vi "final_phd_1.vi"() -> ()   [LabVIEW 2024]
uses:
  <vilib>/Analysis/baseanly.llb/Mean (DBL).vi
  <vilib>/Instr/_visa.llb/VISA Configure Serial Port (Instr).vi
  <vilib>/measure/maspectr.llb/FFT Power Spectrum and PSD for 1 Chan.vi
  <vilib>/Analysis/NI_AALBase.lvlib
  <vilib>/measure/NI_MAPro.lvlib
panel:
  out "Waveform Graph":dbl[](graph)
  out "AI output":u8[](array[numeric])
  in  "Timeout":u32=100
  in  "default name":string
  in  "number":i32=10
  out "Waveform Graph 3":cluster{"f0":dbl, "df":dbl, "magnitude":dbl[]}(graph)={"f0"=0.0, "df"=inf, "magnitude"=[]}
  in  "Signals":waveform(dbl)={"t0"=timestamp(0 s since 1904-01-01), "dt"=0.01, "Y"=[]}
  in  "low cutoff freq":dbl=40.0 format="%0.2f"
  in  "Filter":bool
  in  "Pulse cycle":dbl=1.0
  out "?":dbl(graph)=nan
  in  "milliseconds to wait":u32
  in  "Add Wave 2":bool
  out "Save Status":bool
  in  "Save":bool caption="Save Process"
  out "str_ai_output":string="N.A"
  out "num_sensor_sam_per_cycle":u32=333 caption="Samples/Cycle"
  in  "cbx_sensor_sam_rate":string(combo)="66667" caption="Sample Rate (Hz)"
  in  "num_pulse_samples":u32=500 caption="Samples" max=10000 step=100
  in  "Hidden Controls":T1(tab)
  out "timeout_for_small_data":u32=1000
  out "baud rate":u32=115200
  out "timeout_default":u32=50
  out "termination char":u8
  out "CMD_ID_GET":string
  out "CMD_ID_RUN":string
  out "CMD_ID_NONE":string
  out "CMD_ID_SET":string
  out "CMD_RUN_NONE":string
  out "CMD_RUN_START":string
  out "CMD_RUN_STOP":string
  out "PG_PULSE_NONE":string
  out "PG_PULSE_SQUARE":string
  out "PG_PULSE_SINE":string
  out "RESPONSE_LEN":u32=48
  out "TIM_FREQ":u32=64000000
  out "has_response":bool
  out "ADC_CONVERSION_CYCLES":dbl=8.5
  out "ADC_FREQ":u32=64000000
  out "ADC_SAMPLING_TIME":dbl[](array[numeric])=[2.5, 6.5, 12.5, 24.5, 47.5, 92.5, 247.5, 640.5]
  out "ADC_CLOCK_PRESCALER":u32[](array[numeric])=[1, 2, 4, 6, 8, 10, 12, 16, 32, 64, 128, 256]
  out "sam_rates":cluster{u32, u32, dbl}[](array[cluster])=[{385, 256, 640.5}, {770, 128, 640.5}, {977, 256, 247.5}, {1541, 64, 640.5}, {1953, 128, 247.5}, {2475, 256, 92.5}, {3082, 32, 640.5}, {3906, 64, 247.5}, {4464, 256, 47.5}, {4950, 128, 92.5}, {6163, 16, 640.5}, {7576, 256, 24.5}, {7812, 32, 247.5}, {8218, 12, 640.5}, {8929, 128, 47.5}, {9861, 10, 640.5}, {9901, 64, 92.5}, {11905, 256, 12.5}, {12327, 8, 640.5}, {15152, 128, 24.5}, {15625, 16, 247.5}, {16436, 6, 640.5}, {16667, 256, 6.5}, {17857, 64, 47.5}, {19802, 32, 92.5}, {20833, 12, 247.5}, {22727, 256, 2.5}, {23810, 128, 12.5}, {24653, 4, 640.5}, {25000, 10, 247.5}, {30303, 64, 24.5}, {31250, 8, 247.5}, {33333, 128, 6.5}, {35714, 32, 47.5}, {39604, 16, 92.5}, {41667, 6, 247.5}, {45455, 128, 2.5}, {47619, 64, 12.5}, {49307, 2, 640.5}, {52805, 12, 92.5}, {60606, 32, 24.5}, {62500, 4, 247.5}, {63366, 10, 92.5}, {66667, 64, 6.5}, {71429, 16, 47.5}, {79208, 8, 92.5}, {90909, 64, 2.5}, {95238, 12, 47.5}, {95238, 32, 12.5}, {98613, 1, 640.5}, {105611, 6, 92.5}, {114286, 10, 47.5}, {121212, 16, 24.5}, {125000, 2, 247.5}, {133333, 32, 6.5}, {142857, 8, 47.5}, {158416, 4, 92.5}, {161616, 12, 24.5}, {181818, 32, 2.5}, {190476, 6, 47.5}, {190476, 16, 12.5}, {193939, 10, 24.5}, {242424, 8, 24.5}, {250000, 1, 247.5}, {253968, 12, 12.5}, {266667, 16, 6.5}, {285714, 4, 47.5}, {304762, 10, 12.5}, {316832, 2, 92.5}, {323232, 6, 24.5}, {355556, 12, 6.5}, {363636, 16, 2.5}, {380952, 8, 12.5}, {426667, 10, 6.5}, {484848, 4, 24.5}, {484848, 12, 2.5}, {507937, 6, 12.5}, {533333, 8, 6.5}, {571429, 2, 47.5}, {581818, 10, 2.5}, {633663, 1, 92.5}, {711111, 6, 6.5}, {727273, 8, 2.5}, {761905, 4, 12.5}, {969697, 2, 24.5}, {969697, 6, 2.5}, {1066667, 4, 6.5}, {1142857, 1, 47.5}, {1454545, 4, 2.5}, {1523810, 2, 12.5}, {1939394, 1, 24.5}, {2133333, 2, 6.5}, {2909091, 2, 2.5}, {3047619, 1, 12.5}, {4266667, 1, 6.5}, {5818182, 1, 2.5}]
  out "cbx_sensor_sam_rate_sel_idx":u32=43
  in  "num_senor_read_samples":u32=333 caption="Read Samples" max=10000 step=100
  in  "num_pulse_min_val":dbl caption="Minimum Value (V)" min=0.0 max=1.0 step=0.1
  in  "num_pulse_dutyc":u32=50 caption="Duty Cycle (%)" max=100 step=10
  in  "num_pulse_max_val":dbl=3.0 caption="Maximum Value (V)" min=0.0 max=3.3 step=0.1
  out "?":string
  in  "btn_get":bool
  in  "cbx_pulse_type":string(combo)="1" caption="Type"
  in  "num_pulse_freq":u32=200 caption="Frequency (Hz)" max=2000 step=100
  in  "btn_set":bool
  in  "btn_start_stop":bool
  in  "VISA resource name":refnum<visa-resource-name>="COM10"
  out "read buffer":string
  out "Sensor Signal":dbl[](graph)
  # "NDT COMPACT SYSTEM"
  # "AI Output"
  # "Write Buffer"
  # "Functions Adjustment"
  # "Read Buffer"
  # "Communication"
  # "Settings"
  # "Pulse"
  # "AI OUTPUT"
  # "Sensor"
  # "CT38_koma"
  # "SS400"
  # "Inox201"
  # "Inox304"
  # "Inox316"
  # "AL5052"
  # "Air"
  # "Save data"
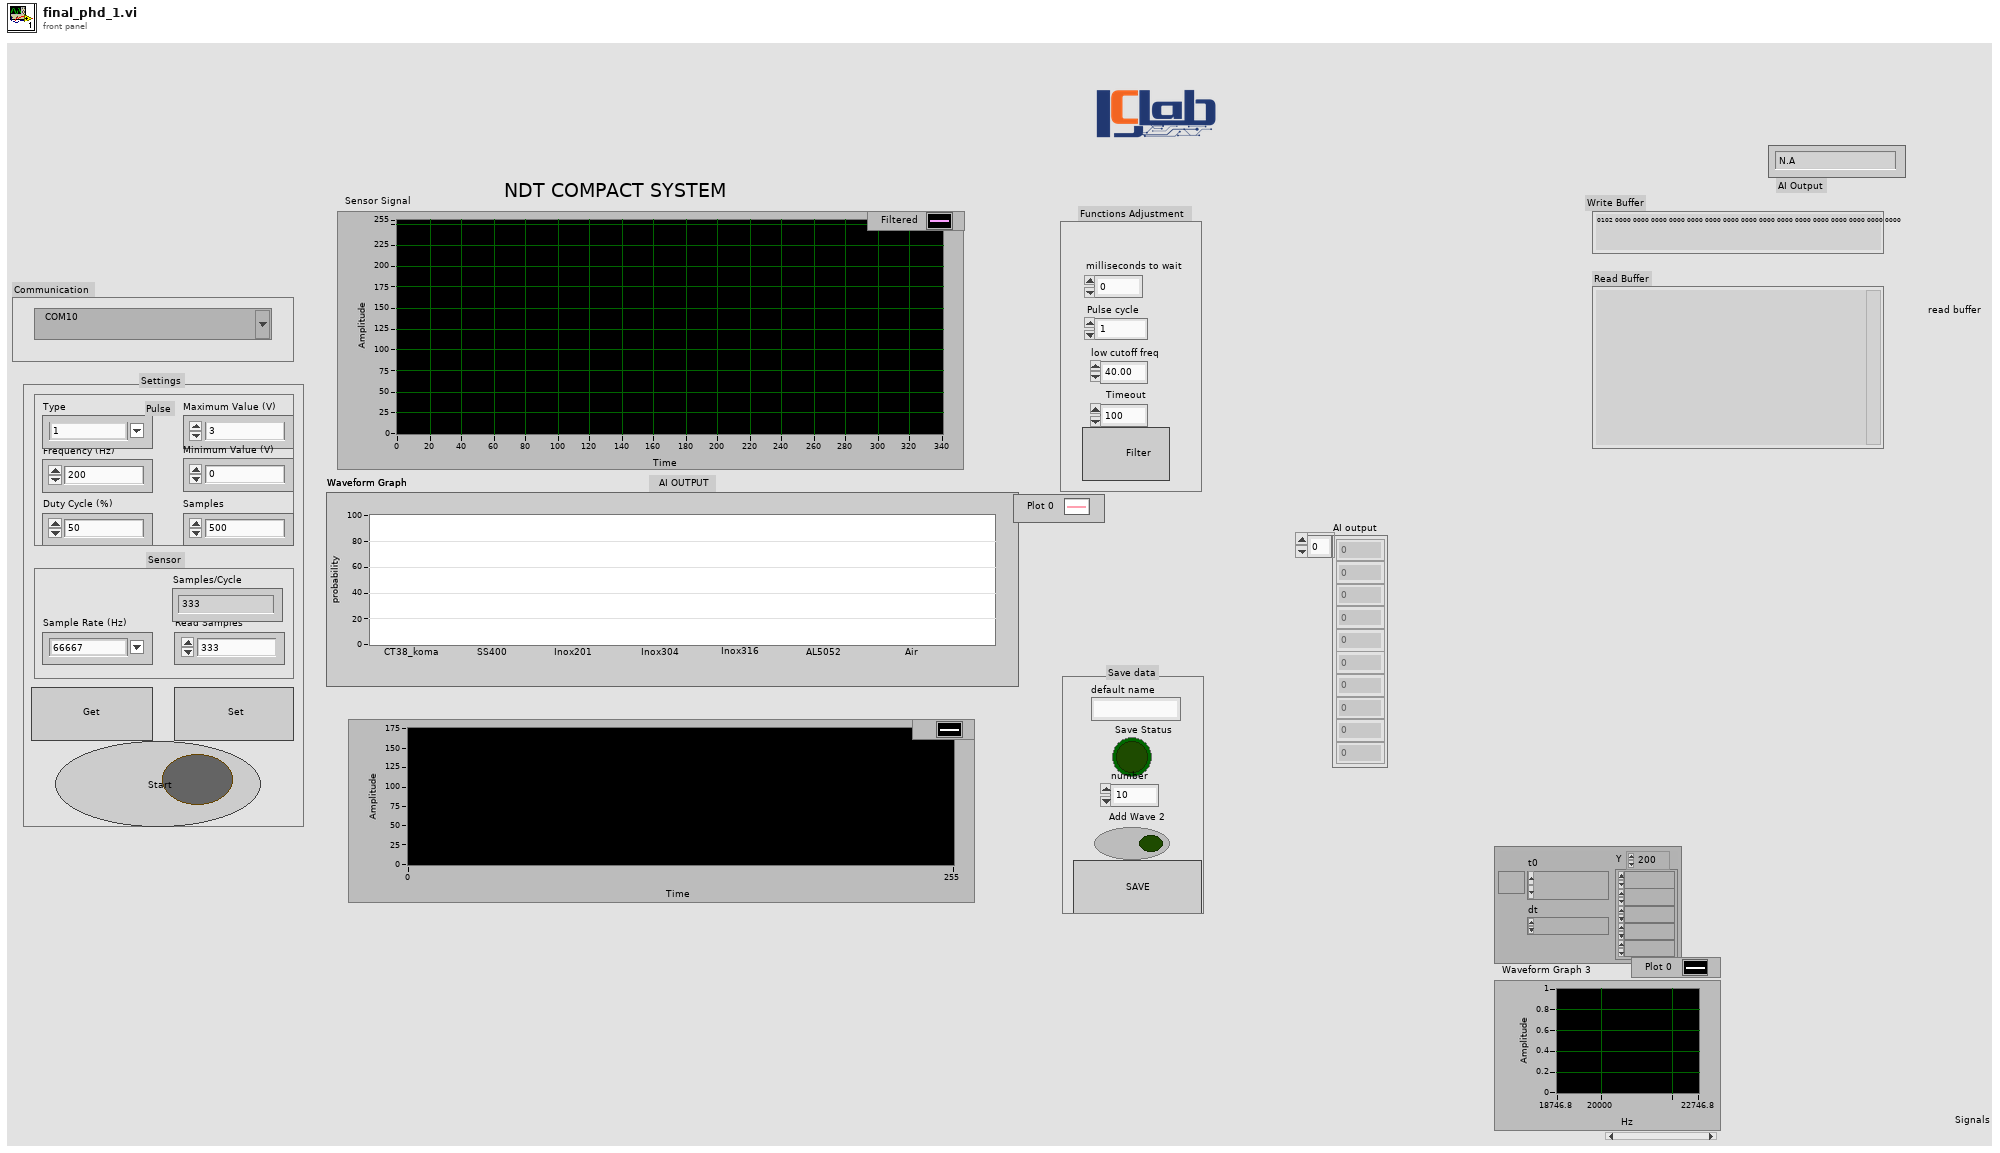
[diagram p1: front panel]
types:
  T1 = enum32{"Page 1", "Page 2", "Page 3", "Page 4", "Page 5"}
  T2 = enum8{"Enabled", "Disabled", "Disabled and Grayed Out"}
  T3 = enum16{"big-endian, network order", "native, host order", "little-endian"}
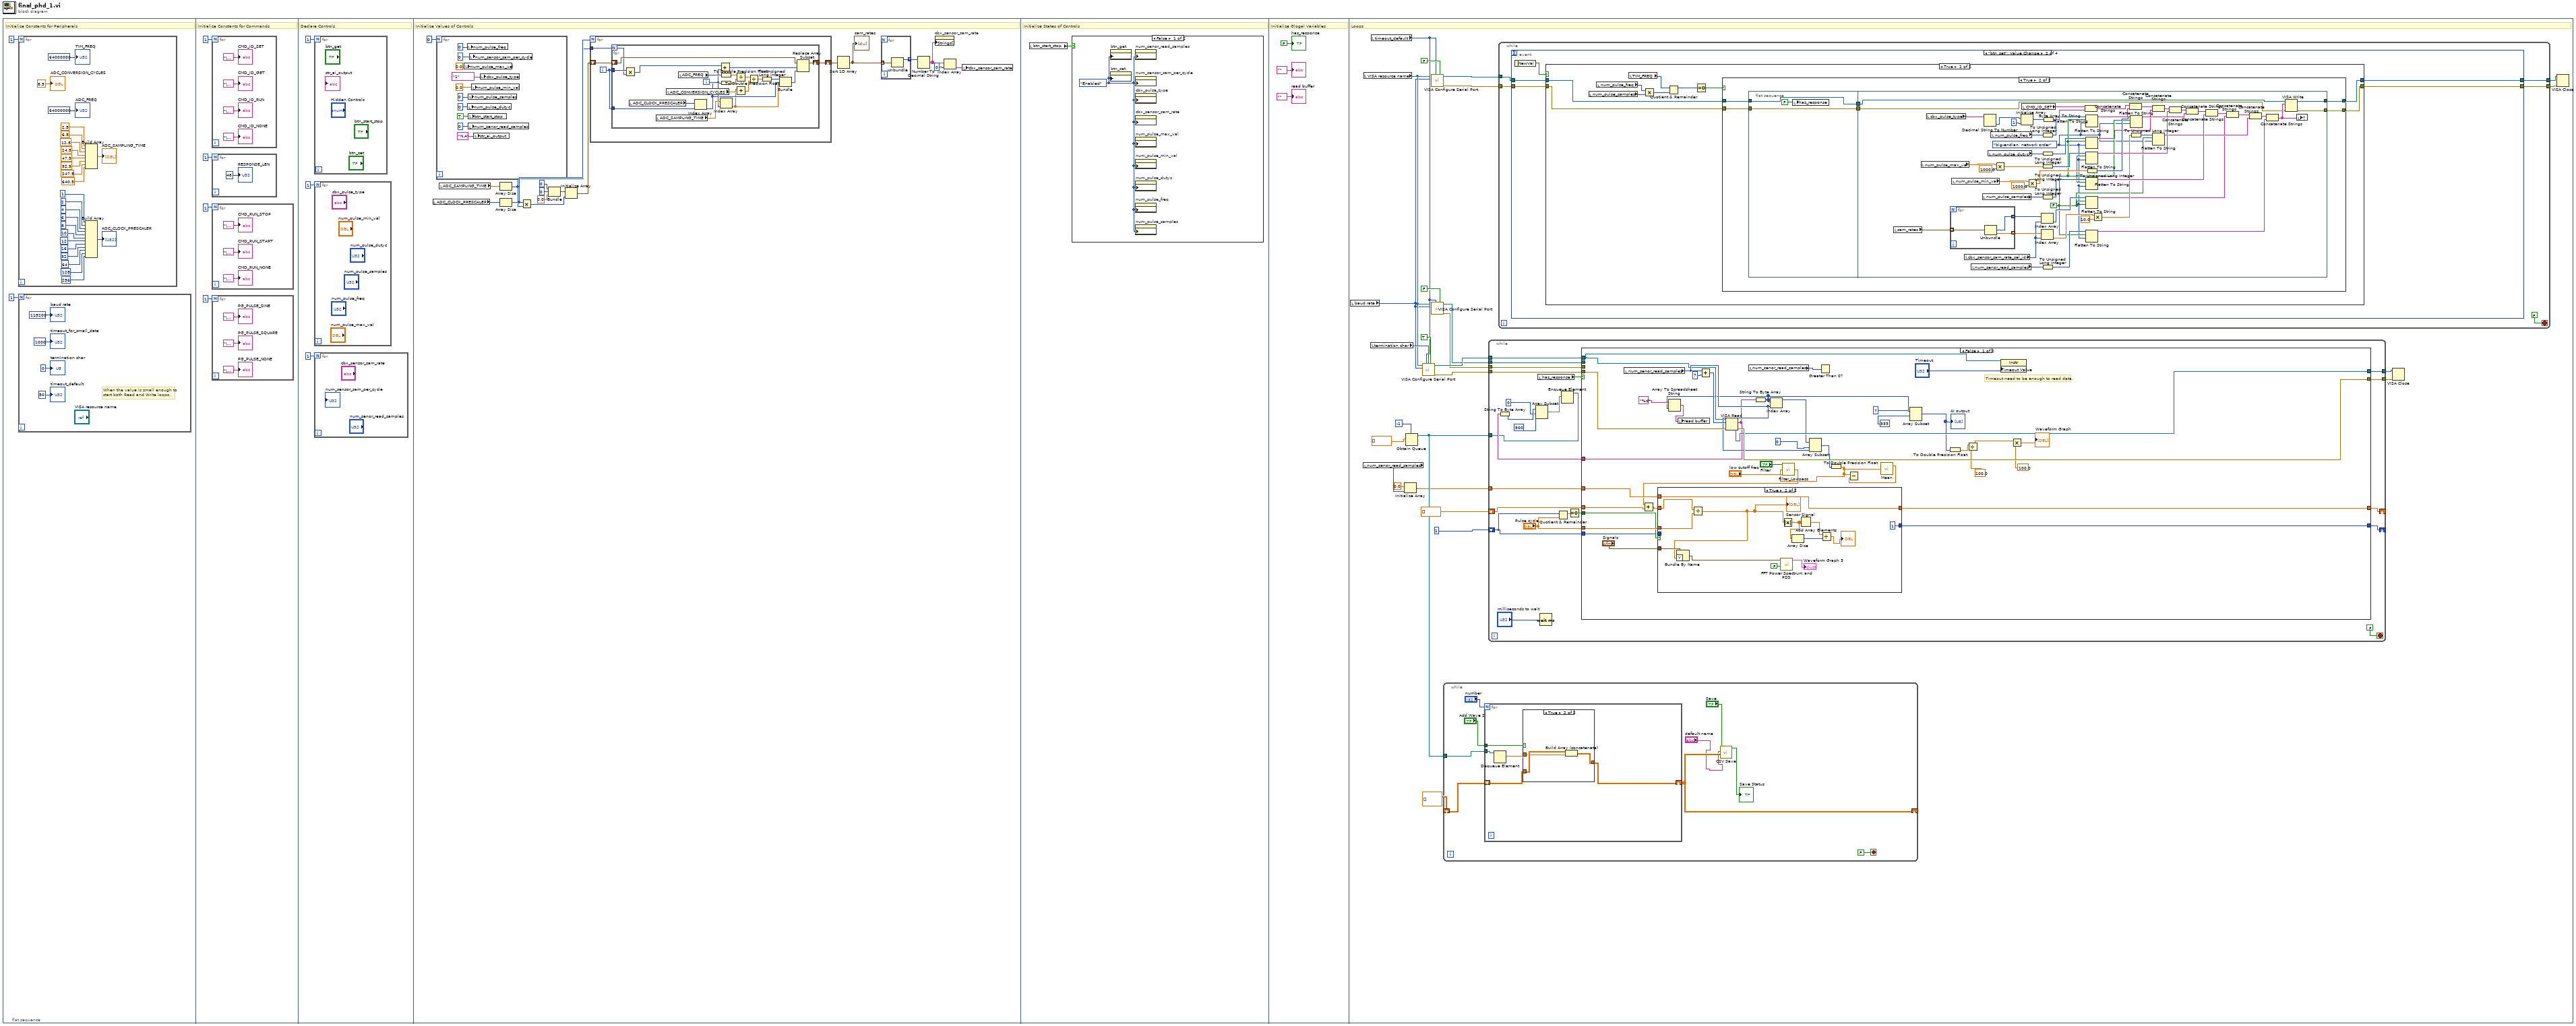
[diagram p0: block diagram]
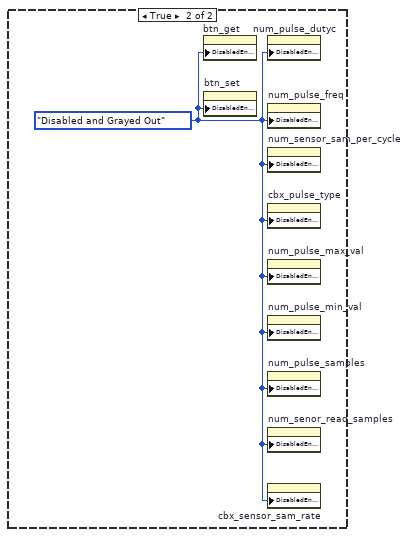
[diagram p2: hidden frame]
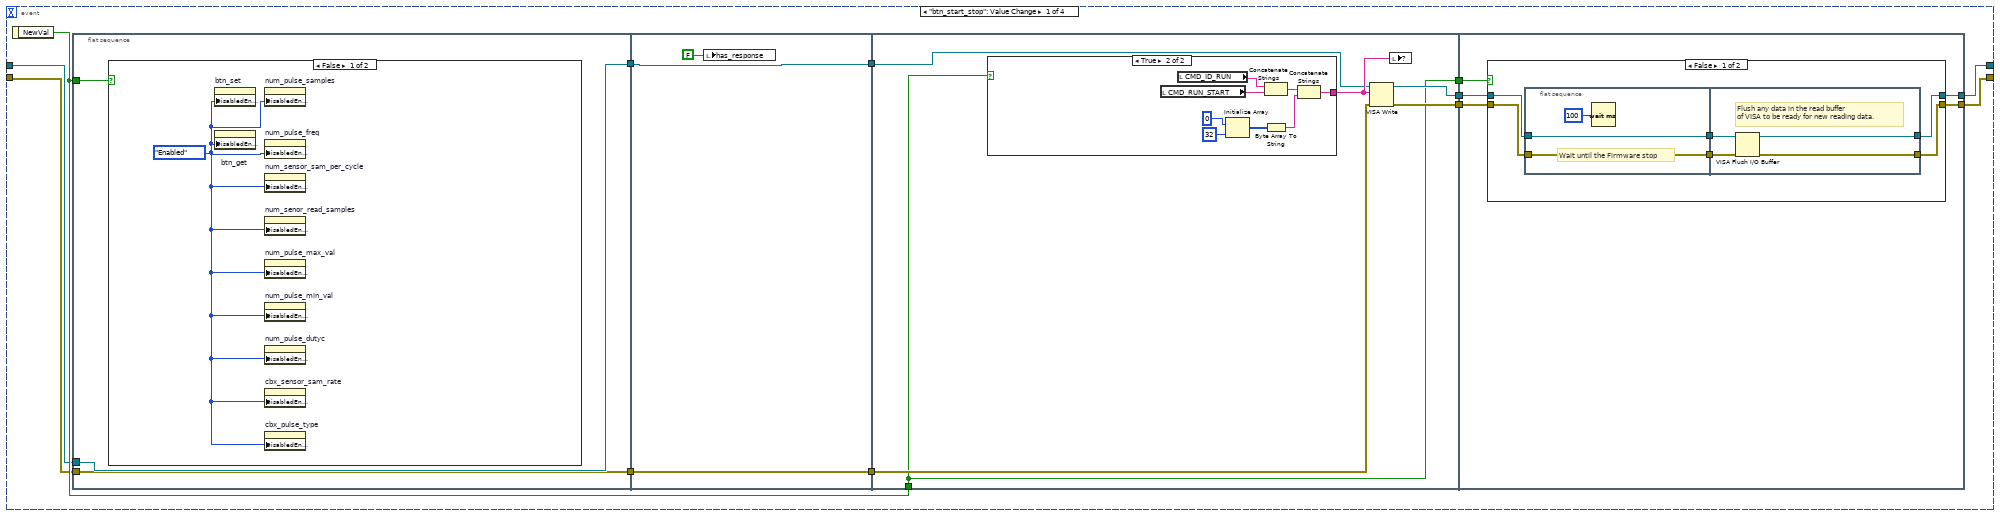
[diagram p4: hidden frame]
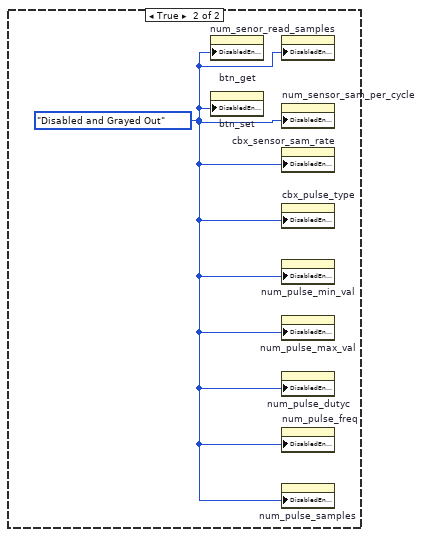
[diagram p5: hidden frame]
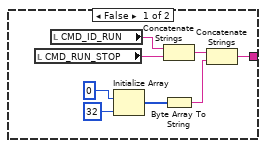
[diagram p6: hidden frame]
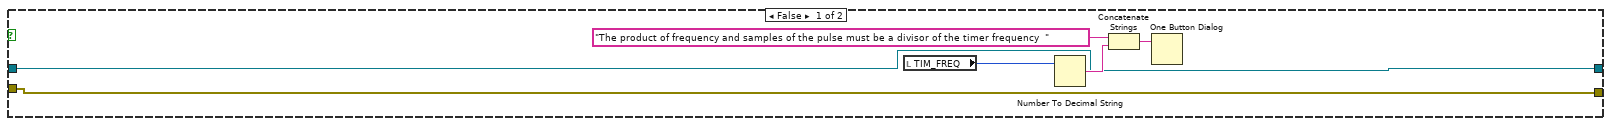
[diagram p9: hidden frame]
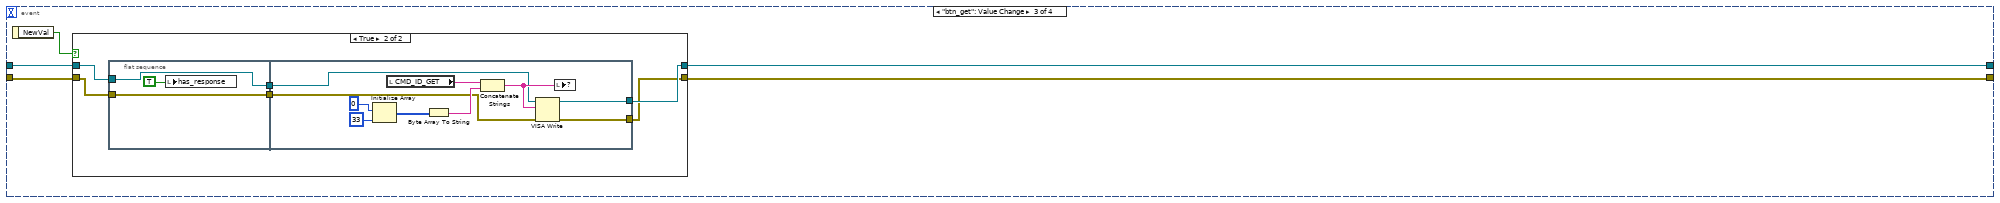
[diagram p10: hidden frame]
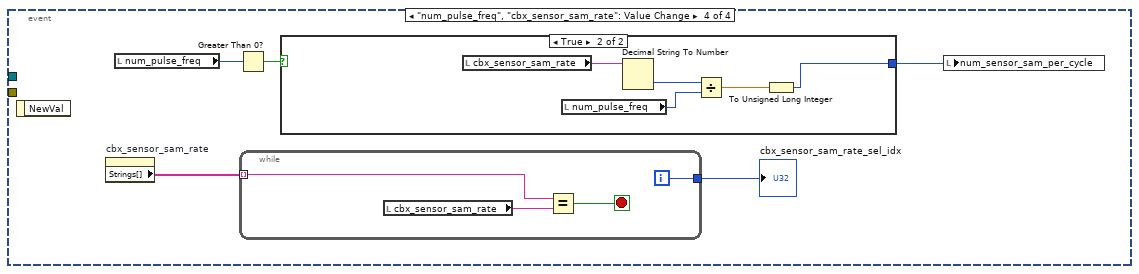
[diagram p12: hidden frame]
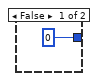
[diagram p13: hidden frame]
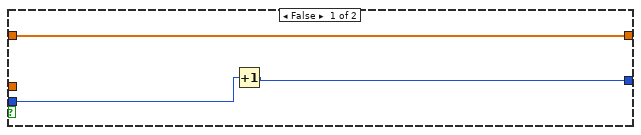
[diagram p14: hidden frame]
diagram:
  n1 = flat-sequence {
    frame #0 {
      # "Initialize Constants for Peripherals"
      n2 = for {
        N: 1 -> [_]
        n3 = Build Array(2.5 ("element"), 6.5 ("element"), 12.5 ("element"), 24.5 ("element"), 47.5 ("element"), 92.5 ("element"), 247.5 ("element"), 640.5 ("element")) -> (→"ADC_SAMPLING_TIME":dbl[])
        n4 = Build Array(u32 1 ("element"), u32 2 ("element"), u32 4 ("element"), u32 6 ("element"), u32 8 ("element"), u32 10 ("element"), u32 12 ("element"), u32 16 ("element"), u32 32 ("element"), u32 64 ("element"), u32 128 ("element"), u32 256 ("element")) -> (→"ADC_CLOCK_PRESCALER":u32[])
        "ADC_CONVERSION_CYCLES" <- 8.5
        "ADC_FREQ" <- 64000000
        "TIM_FREQ" <- 64000000
      }
      n5 = for {
        N: 1 -> [_]
        # "When the value is small enough to\nstart both Read and Write loops."
        "baud rate" <- u32 115200 ("baud rate (9600)")
        "timeout_default" <- u32 50 ("timeout (10sec)")
        "termination char" <- u8 0 ("termination char\n(0xA = '\\n' = LF)")
        "timeout_for_small_data" <- u32 1000 ("timeout_default 2")
      }
    }
    frame #1 {
      # "Initialize Constants for Commands"
      n6 = for {
        N: 1 -> [_]
        "CMD_ID_NONE" <- "\u0000"
        "CMD_ID_RUN" <- "\u0001"
        "CMD_ID_GET" <- "\u0002"
        "CMD_ID_SET" <- "\u0003"
      }
      n7 = for {
        N: 1 -> [_]
        "RESPONSE_LEN" <- 48
      }
      n8 = for {
        N: 1 -> [_]
        "CMD_RUN_NONE" <- "\u0000"
        "CMD_RUN_START" <- "\u0001"
        "CMD_RUN_STOP" <- "\u0002"
      }
      n9 = for {
        N: 1 -> [_]
        "PG_PULSE_NONE" <- "\u0000"
        "PG_PULSE_SQUARE" <- "\u0001"
        "PG_PULSE_SINE" <- "\u0002"
      }
    }
    frame #2 {
      # "Declare Controls"
      n10 = for {
        N: 1 -> [_]
      }
      n11 = for {
        N: 1 -> [_]
      }
      n12 = for {
        N: 1 -> [_]
      }
    }
    frame #3 {
      # "Initialize Values of Controls"
      n13 = local read "ADC_CLOCK_PRESCALER"() -> (w60:u32[])
      n14 = for {
        N: 0 -> [_]
        n15 = local write "num_pulse_max_val"(0.0 ("num_pulse_amp")) -> ()
        n16 = local write "num_pulse_freq"(u32 0 ("num_pulse_freq")) -> ()
        n17 = local write "num_pulse_dutyc"(u32 0 ("num_pulse_dutyc")) -> ()
        n18 = local write "num_pulse_samples"(u32 0 ("num_pulse_samples")) -> ()
        n19 = local write "btn_start_stop"(TRUE ("btn_start_stop")) -> ()
        n20 = local write "num_senor_read_samples"(u32 0 ("num_read_samples")) -> ()
        n21 = local write "num_sensor_sam_per_cycle"(u32 0 ("num_sensor_sam_per_cycle")) -> ()
        n22 = local write "num_pulse_min_val"(0.0 ("num_pulse_amp_offset")) -> ()
        n23 = local write "str_ai_output"("N.A" ("str_ai_result")) -> ()
        n24 = local write "cbx_pulse_type"("1" ("cbx_pulse_type")) -> ()
      }
      n25 = local read "ADC_SAMPLING_TIME"() -> (w59:dbl[])
      n26 = Array Size(array=w59) -> (size(s)=w55:i32)
      n27 = Array Size(array=w60) -> (size(s)=w56:i32)
      n28 = Multiply(x=w56, y=w55) -> (x*y=w57:i32)
      n29 = Bundle(u32 0, u32 0, 0.0) -> (w61:cluster{u32, u32, dbl})  [unwired: 1 in]
      n30 = Initialize Array(w61, w57) -> (w54:cluster{u32, u32, dbl}[])
      n31 = for {
        N: w56 -> [_]
        tunnel: w55 -> [w72]
        shift-right: [w70] -> w58
        shift-left: w54 -> [w71]
        i -> [w69]
        n32 = for {
          N: w72 -> [w81]
          tunnel: w69 -> [w90]
          shift-right: [w78] -> w70
          shift-left: w71 -> [w84]
          tunnel: w69 -> [w82]
          i -> [w80]
          n33 = Multiply(x=w82, y=w81) -> (x*y=w83:i32)
          n34 = local read "ADC_CLOCK_PRESCALER"() -> (w91:u32[])
          n35 = local read "ADC_SAMPLING_TIME"() -> (w92:dbl[])
          n36 = local read "ADC_CONVERSION_CYCLES"() -> (w93:dbl)
          n37 = local read "ADC_FREQ"() -> (w86:u32)
          n38 = Index Array(array=w91, index=w90) -> (element=w74:u32)
          n39 = Add(x=w83, y=w80) -> (x+y=w79:i32)
          n40 = To Double Precision Float(number=w86) -> (double precision float=w85:dbl)
          n41 = To Double Precision Float(number=w74) -> (double precision float=w87:dbl)
          n42 = Index Array(array=w92, index=w80) -> (element=w73:dbl)
          n43 = Divide(x=w85, y=w87) -> (x/y=w89:dbl)
          n44 = Add(x=w93, y=w73) -> (x+y=w88:dbl)
          n45 = Divide(x=w89, y=w88) -> (x/y=w76:dbl)
          n46 = To Unsigned Long Integer(number=w76) -> (unsigned 32bit integer=w75:u32)
          n47 = Bundle(w75, "element"=w74, "element"=w73) -> (w77:cluster{u32, "element":u32, "element":dbl})  [unwired: 1 in]
          n48 = Replace Array Subset(array=w84, new element=w77, index=w79) -> (w78:cluster{u32, u32, dbl}[])
        }
      }
      n49 = Sort 1D Array(array=w58) -> (sorted array=w62:cluster{u32, u32, dbl}[])
      "sam_rates" <- w62
      n50 = for {
        tunnel: w62 -> [w68] mode=indexing
        tunnel: [w67] -> w63 mode=indexing
        n51 = Unbundle(w68) -> (w67:u32)  [unwired: 2 out]
      }
      n52 = Number To Decimal String(number=w63) -> (decimal integer string=w64:string[])  [unwired: 1 in]
      n53 = property on="cbx_sensor_sam_rate" class="CmbBox"("Strings[]"=w64) -> ()  [unwired: 2 in, 2 out]
      n54 = Index Array(array=w64, index=0) -> (element=w65:string)
      n55 = local write "cbx_sensor_sam_rate"(w65) -> ()
    }
    frame #4 {
      # "Initialize States of Controls"
      n56 = local read "btn_start_stop"() -> (w104:bool)
      n57 = case shown="False" w104 {
        frame False {
          w105 = T2."Enabled" ("Disabled")
          n58 = property on="btn_get" class="Bool (strict)"("DisabledEnum"=w105) -> ()  [unwired: 2 in, 2 out]
          n59 = property on="btn_set" class="Bool (strict)"("DisabledEnum"=w105) -> ()  [unwired: 2 in, 2 out]
          n60 = property on="num_senor_read_samples" class="DigNum (strict)"("DisabledEnum"=w105) -> ()  [unwired: 2 in, 2 out]
          n61 = property on="num_sensor_sam_per_cycle" class="DigNum (strict)"("DisabledEnum"=w105) -> ()  [unwired: 2 in, 2 out]
          n62 = property on="cbx_pulse_type" class="CmbBox"("DisabledEnum"=w105) -> ()  [unwired: 2 in, 2 out]
          n63 = property on="cbx_sensor_sam_rate" class="CmbBox"("DisabledEnum"=w105) -> ()  [unwired: 2 in, 2 out]
          n64 = property on="num_pulse_max_val" class="DigNum (strict)"("DisabledEnum"=w105) -> ()  [unwired: 2 in, 2 out]
          n65 = property on="num_pulse_min_val" class="DigNum (strict)"("DisabledEnum"=w105) -> ()  [unwired: 2 in, 2 out]
          n66 = property on="num_pulse_dutyc" class="DigNum (strict)"("DisabledEnum"=w105) -> ()  [unwired: 2 in, 2 out]
          n67 = property on="num_pulse_freq" class="DigNum (strict)"("DisabledEnum"=w105) -> ()  [unwired: 2 in, 2 out]
          n68 = property on="num_pulse_samples" class="DigNum (strict)"("DisabledEnum"=w105) -> ()  [unwired: 2 in, 2 out]
        }
        frame True {
          w106 = T2."Disabled and Grayed Out" ("Disabled")
          n69 = property on="btn_get" class="Bool (strict)"("DisabledEnum"=w106) -> ()  [unwired: 2 in, 2 out]
          n70 = property on="btn_set" class="Bool (strict)"("DisabledEnum"=w106) -> ()  [unwired: 2 in, 2 out]
          n71 = property on="num_pulse_dutyc" class="DigNum (strict)"("DisabledEnum"=w106) -> ()  [unwired: 2 in, 2 out]
          n72 = property on="num_pulse_freq" class="DigNum (strict)"("DisabledEnum"=w106) -> ()  [unwired: 2 in, 2 out]
          n73 = property on="num_sensor_sam_per_cycle" class="DigNum (strict)"("DisabledEnum"=w106) -> ()  [unwired: 2 in, 2 out]
          n74 = property on="cbx_pulse_type" class="CmbBox"("DisabledEnum"=w106) -> ()  [unwired: 2 in, 2 out]
          n75 = property on="num_pulse_max_val" class="DigNum (strict)"("DisabledEnum"=w106) -> ()  [unwired: 2 in, 2 out]
          n76 = property on="num_pulse_min_val" class="DigNum (strict)"("DisabledEnum"=w106) -> ()  [unwired: 2 in, 2 out]
          n77 = property on="num_pulse_samples" class="DigNum (strict)"("DisabledEnum"=w106) -> ()  [unwired: 2 in, 2 out]
          n78 = property on="num_senor_read_samples" class="DigNum (strict)"("DisabledEnum"=w106) -> ()  [unwired: 2 in, 2 out]
          n79 = property on="cbx_sensor_sam_rate" class="CmbBox"("DisabledEnum"=w106) -> ()  [unwired: 2 in, 2 out]
        }
      }
    }
    frame #5 {
      # "Initialize Glogal Variables"
      "?" <- "" ("write buffer")
      "read buffer" <- "" ("read buffer")
      "has_response" <- FALSE
    }
    frame #6 {
      # "Loops"
      n80 = local read "baud rate"() -> (w119:u32)
      n81 = local read "num_senor_read_samples"() -> (w112:u32)
      n82 = local read "VISA resource name"() -> (w120:refnum<visa-resource-name>)
      n83 = local read "termination char"() -> (w132:u8)
      n84 = local read "timeout_default"() -> (w121:u32)
      n85 = Initialize Array(0.0 ("element"), w112) -> (w111:dbl[])
      n86 = Obtain Queue(max queue size (-1, unlimited)=-1, element data type=dbl[] []) -> (queue out=w116:refnum<queue>)  [unwired: 3 in, 2 out]
      n87 = call-poly "VISA Configure Serial Port"("VISA resource name"=w120, "timeout (10sec)"=w121, "termination char\n(0xA = '\\n' = LF)"=w132, "Enable Termination\nChar (T)"=TRUE ("Enable Termination\nChar (T)"), "baud rate (9600)"=w119) -> ("VISA resource name out"=w133:refnum<visa-resource-name>, "error out"=w127:errorcluster)  [unwired: 9 in]
      n88 = call-poly "VISA Configure Serial Port"("VISA resource name"=w120, "timeout (10sec)"=w121, "Enable Termination\nChar (T)"=FALSE ("Enable Termination\nChar (T)"), "baud rate (9600)"=w119) -> ("VISA resource name out"=w124:refnum<visa-resource-name>, "error out"=w123:errorcluster)  [unwired: 10 in]
      n89 = call-poly "VISA Configure Serial Port"("VISA resource name"=w120, "timeout (10sec)"=w121, "Enable Termination\nChar (T)"=FALSE ("Enable Termination\nChar (T)"), "baud rate (9600)"=w119) -> ("VISA resource name out"=w125:refnum<visa-resource-name>, "error out"=w126:errorcluster)  [unwired: 10 in]
      n90 = while {
        tunnel: w116 -> [w142]
        shift-right: [w139] -> _
        shift-left: dbl[][] [] -> [w140]
        stop <- FALSE stop-if-true
        n91 = for {
          N: "number" -> [_]
          tunnel: "Add Wave 2" -> [w149]
          shift-right: [w145] -> w139
          shift-left: w140 -> [w148]
          tunnel: w142 -> [w147]
          n92 = Dequeue Element(queue=w147) -> (element=w146:dbl[])  [unwired: 2 in, 3 out]
          n93 = case shown="True" w149 {
            tunnel: w146 -> [_ w152]
            tunnel: [w150 w151] -> w145
            tunnel: w148 -> [w150 w153]
            frame False {
            }
            frame True {
              n94 = Build Array (concatenate)(w153, w152) -> (w151:dbl[][])
            }
          }
        }
        n95 = call "CSV Save.vi"("Array"=w139, "default name"="default name", "Save Button"="Save") -> ("Save Status"=→"Save Status":bool)  [unwired: 8 in]
      }
      n96 = while {
        tunnel: w133 -> [w371]
        tunnel: w127 -> [w372]
        tunnel: [w370] -> w134
        tunnel: [w369] -> w135
        tunnel: w125 -> [w368]
        tunnel: w126 -> [w367]
        tunnel: w116 -> [w360]
        shift-right: [w354] -> _
        shift-left: dbl[] [] -> [w355]
        shift-right: [w353] -> _
        shift-left: 1 ("max queue size (-1, unlimited)") -> [w352]
        tunnel: w111 -> [w351]
        stop <- FALSE stop-if-true
        n97 = local read "has_response"() -> (w373:bool)
        n98 = Wait (ms)(milliseconds to wait="milliseconds to wait") -> ()  [unwired: 1 out]
        n99 = Quotient & Remainder(x=w352, y="Pulse cycle") -> (x-y*floor(x/y)=w356:dbl)  [unwired: 1 out]
        n100 = Equal To 0?(x=w356) -> (x = 0?=w358:bool)
        n101 = case shown="False" w373 {
          tunnel: w372 -> [w409 _]
          tunnel: w371 -> [w402 _]
          tunnel: [w408 w432] -> w369
          tunnel: [w407 w434] -> w370
          tunnel: w368 -> [_ w430]
          tunnel: w367 -> [_ w435]
          tunnel: [w401 w429] -> w361
          tunnel: w358 -> [w398 _]
          tunnel: "Pulse cycle" -> [w399 _]
          tunnel: w355 -> [w397 w427]
          tunnel: [w395 w427] -> w354
          tunnel: w352 -> [w394 w428]
          tunnel: [w393 w428] -> w353
          tunnel: w351 -> [w392 _]
          frame False {
            # "Timeout need to be enough to read data."
            n102 = local read "num_senor_read_samples"() -> (w404:u32)
            n103 = Add(x=w404, y=u32 7) -> (x+y=w405:u32)
            n104 = VISA Read(VISA resource name=w402, byte count=w405, error in (no error)=w409) -> (VISA resource name out=w407:refnum<visa-resource-name>, read buffer=w401:string, error out=w408:errorcluster)  [unwired: 1 out]
            n105 = local read "num_senor_read_samples"() -> (w403:u32)
            n106 = String To Byte Array(string=w401) -> (unsigned byte array=w382:u8[])
            n107 = Array To Spreadsheet String(array=w382, 3:"%d" ("format string")) -> (spreadsheet string=w383:string)  [unwired: 1 in]
            n108 = local write "read buffer"(w383) -> ()
            n109 = Index Array(array=w382, index=w404) -> ()  [unwired: 1 out]
            n110 = Array Subset(array=w382, index=0, length=w404) -> (w400:u8[])
            n111 = Greater Than 0?(x=w403) -> ()  [unwired: 1 out]
            n112 = To Double Precision Float(number=w400) -> (double precision float=w387:dbl[])
            n113 = call "Filter_Lowpass.vi"("Filter"="Filter", "Pulse signal in"=w387, "low cutoff freq: fl"="low cutoff freq") -> ("Signal out"=w388:dbl[])  [unwired: 6 in]
            n114 = Add(x=w388, y=w397) -> (x+y=w396:dbl[])
            n115 = case shown="True" w398 {
              tunnel: w399 -> [_ w422]
              tunnel: w396 -> [w413 w421]
              tunnel: [w413 w419] -> w395
              tunnel: w394 -> [w412 _]
              tunnel: [w411 1] -> w393
              tunnel: w392 -> [_ w419]
              tunnel: "Signals" -> [_ w417]
              frame False {
                n116 = Increment(x=w412) -> (x+1=w411:i32)
              }
              frame True {
                n117 = Divide(x=w421, y=w422) -> (x/y=w414:dbl[])
                "Sensor Signal" <- w414
                n118 = Bundle By Name(cluster=w417, "Y"=w414) -> (w416:waveform(dbl))
                n119 = call-poly <vilib>:"FFT Power Spectrum and PSD.vi"("dB On (F)"=FALSE, "time signal"=w416) -> ("Power Spectrum / PSD"=→"Waveform Graph 3":cluster{"f0":dbl, "df":dbl, "magnitude":dbl[]})  [unwired: 6 in, 3 out]
                n120 = Absolute Value(x=w414) -> (abs(x)=w423:dbl[])
                n121 = Array Size(array=w423) -> (size(s)=w425:i32)
                n122 = Add Array Elements(numeric array=w423) -> (sum=w426:dbl)
                n123 = Divide(x=w426, y=w425) -> (x/y=→"?":dbl)
              }
            }
            n124 = call-poly <vilib>:"Mean.vi"("X"=w387) -> ("mean"=w389:dbl)  [unwired: 1 out]
            n125 = Subtract(x=w387, y=w389) -> ()  [unwired: 1 out]
            n126 = Array Subset(array=w382, index=333, length=7) -> (w379:u8[])
            "AI output" <- w379
            n127 = To Double Precision Float(number=w379) -> (double precision float=w378:dbl[])
            n128 = Divide(x=w378, y=100.0) -> (x/y=w375:dbl[])
            n129 = property class="Instr"(reference=w402, "General Settings:Timeout Value"="Timeout") -> ()  [unwired: 1 in, 2 out]
            n130 = Multiply(x=w375, y=100.0) -> (x*y=→"Waveform Graph":dbl[])
          }
          frame True {
            n131 = flat-sequence {
              tunnel: w430 -> [w444]
              tunnel: w435 -> [w443]
              tunnel: [w442] -> w433
              tunnel: [w441] -> w431
              tunnel: [w436] -> w429
              tunnel: [w508] -> w434
              tunnel: w433 -> [w508]
              tunnel: [w507] -> w432
              tunnel: w431 -> [w507]
              frame #0 {
                n132 = local read "RESPONSE_LEN"() -> (w446:u32)
                n133 = local read "CMD_ID_GET"() -> (w438:string)
                n134 = VISA Read(VISA resource name=w444, byte count=w446, error in (no error)=w443) -> (VISA resource name out=w442:refnum<visa-resource-name>, read buffer=w436:string, error out=w441:errorcluster)  [unwired: 1 out]
                n135 = local write "read buffer"(w436) -> ()
                n136 = String To Byte Array(string=w438) -> (unsigned byte array=w440:u8[])
                n137 = String To Byte Array(string=w436) -> (unsigned byte array=w449:u8[])
                n138 = Index Array(array=w449, index=0) -> (element=w447:u8)
                n139 = Index Array(array=w440, index=0) -> (element=w437:u8)
                n140 = Equal?(x=w447, y=w437) -> (x = y?=w448:bool)
                n141 = case shown="True" w448 {
                  tunnel: w449 -> [_ w506]
                  tunnel: w436 -> [_ w466]
                  frame False {
                  }
                  frame True {
                    w465 = FALSE ("data includes array or string size? (T)")
                    w464 = T3."big-endian, network order" ("byte order (0:big-endian, network order)")
                    n142 = Index Array(array=w506, index=1) -> (element=w488:u8)
                    n143 = String Subset(string=w466, offset (0)=18, length (rest)=4 ("length (rest)")) -> (substring=w486:string)
                    n144 = String Subset(string=w466, offset (0)=14, length (rest)=4 ("length (rest)")) -> (substring=w489:string)
                    n145 = String Subset(string=w466, offset (0)=10, length (rest)=4 ("length (rest)")) -> (substring=w496:string)
                    n146 = String Subset(string=w466, offset (0)=30, length (rest)=4 ("length (rest)")) -> (substring=w483:string)
                    n147 = String Subset(string=w466, offset (0)=22, length (rest)=4 ("length (rest)")) -> (substring=w471:string)
                    n148 = String Subset(string=w466, offset (0)=26, length (rest)=4 ("length (rest)")) -> (substring=w468:string)
                    n149 = Number To Decimal String(number=w488) -> (decimal integer string=w474:string)  [unwired: 1 in]
                    n150 = property on="cbx_pulse_type" class="CmbBox"("Val(Sgnl)"=w474) -> ()  [unwired: 2 in, 2 out]
                    n151 = String Subset(string=w466, offset (0)=2, length (rest)=4 ("length (rest)")) -> (substring=w498:string)
                    n152 = String Subset(string=w466, offset (0)=6, length (rest)=4 ("length (rest)")) -> (substring=w497:string)
                    n153 = To Unsigned Long Integer(number=u32 0) -> (unsigned 32bit integer=w463:u32)
                    n154 = local read "ADC_FREQ"() -> (w460:u32)
                    n155 = Unflatten From String(type=w463, binary string=w486, data includes array or string size? (T)=w465, byte order (0:big-endian, network order)=w464) -> (value=w475:u32)  [unwired: 1 in, 2 out]
                    n156 = Unflatten From String(type=w463, binary string=w489, data includes array or string size? (T)=w465, byte order (0:big-endian, network order)=w464) -> (value=w493:u32)  [unwired: 1 in, 2 out]
                    n157 = Unflatten From String(type=w463, binary string=w483, data includes array or string size? (T)=w465, byte order (0:big-endian, network order)=w464) -> (value=w477:u32)  [unwired: 1 in, 2 out]
                    n158 = Unflatten From String(type=w463, binary string=w471, data includes array or string size? (T)=w465, byte order (0:big-endian, network order)=w464) -> (value=w457:u32)  [unwired: 1 in, 2 out]
                    n159 = Unflatten From String(type=w463, binary string=w468, data includes array or string size? (T)=w465, byte order (0:big-endian, network order)=w464) -> (value=w462:u32)  [unwired: 1 in, 2 out]
                    n160 = Unflatten From String(type=w463, binary string=w496, data includes array or string size? (T)=w465, byte order (0:big-endian, network order)=w464) -> (value=w495:u32)  [unwired: 1 in, 2 out]
                    n161 = Unflatten From String(type=w463, binary string=w498, data includes array or string size? (T)=w465, byte order (0:big-endian, network order)=w464) -> (value=w480:u32)  [unwired: 1 in, 2 out]
                    n162 = Unflatten From String(type=w463, binary string=w497, data includes array or string size? (T)=w465, byte order (0:big-endian, network order)=w464) -> (value=w479:u32)  [unwired: 1 in, 2 out]
                    n163 = local read "ADC_CONVERSION_CYCLES"() -> (w456:dbl)
                    n164 = property on="num_pulse_samples" class="DigNum (strict)"("Val(Sgnl)"=w475) -> ()  [unwired: 2 in, 2 out]
                    n165 = property on="num_senor_read_samples" class="DigNum (strict)"("Val(Sgnl)"=w477) -> ()  [unwired: 2 in, 2 out]
                    n166 = property on="num_pulse_freq" class="DigNum (strict)"("Val(Sgnl)"=w480) -> ()  [unwired: 2 in, 2 out]
                    n167 = property on="num_pulse_dutyc" class="DigNum (strict)"("Val(Sgnl)"=w479) -> ()  [unwired: 2 in, 2 out]
                    n168 = To Double Precision Float(number=w460) -> (double precision float=w459:dbl)
                    n169 = To Double Precision Float(number=w457) -> (double precision float=w458:dbl)
                    n170 = To Double Precision Float(number=w462) -> (double precision float=w467:dbl)
                    n171 = Divide(x=w493, y=1000.0) -> (x/y=w476:dbl)
                    n172 = Divide(x=w495, y=1000.0) -> (x/y=w478:dbl)
                    n173 = Divide(x=w459, y=w458) -> (x/y=w454:dbl)
                    n174 = Divide(x=w467, y=10.0) -> (x/y=w455:dbl)
                    n175 = property on="num_pulse_min_val" class="DigNum (strict)"("Val(Sgnl)"=w476) -> ()  [unwired: 2 in, 2 out]
                    n176 = property on="num_pulse_max_val" class="DigNum (strict)"("Val(Sgnl)"=w478) -> ()  [unwired: 2 in, 2 out]
                    n177 = Add(x=w456, y=w455) -> (x+y=w453:dbl)
                    n178 = Divide(x=w454, y=w453) -> (x/y=w452:dbl)
                    n179 = To Unsigned Long Integer(number=w452) -> (unsigned 32bit integer=w451:u32)
                    n180 = Number To Decimal String(number=w451) -> (decimal integer string=w450:string)  [unwired: 1 in]
                    n181 = property on="cbx_sensor_sam_rate" class="CmbBox"("Val(Sgnl)"=w450) -> ()  [unwired: 2 in, 2 out]
                  }
                }
              }
              frame #1 {
                n182 = local write "has_response"(FALSE ("IS_RESPONSE")) -> ()
              }
            }
          }
        }
        n183 = String To Byte Array(string=w361) -> (unsigned byte array=w364:u8[])
        n184 = Array Subset(array=w364, index=0, length=500) -> (w365:u8[])
        n185 = Enqueue Element(queue=w360, element=w365) -> ()  [unwired: 2 in, 3 out]
      }
      n186 = while {
        tunnel: [w158] -> w129
        tunnel: [w157] -> w128
        tunnel: w124 -> [w154]
        tunnel: w123 -> [w155]
        stop <- FALSE stop-if-true
        n187 = event shown="[1] \"btn_set\": Value Change" {
          selector: _ -> [_ _ _ _]
          dyn-events: _ -> [_ _ _ _]
          timeout: _ -> [_ _ _ _]
          tunnel: [w160 w224 w311 _] -> w158
          tunnel: [w159 w223 w310 _] -> w157
          tunnel: w155 -> [w164 w221 w313 _]
          tunnel: w154 -> [w165 w222 w312 _]
          event "btn_start_stop": Value Change {
            n188 = event-data() -> ("NewVal"=w170:bool)  [unwired: 1 in]
            n189 = flat-sequence {
              tunnel: w170 -> [w173]
              tunnel: w165 -> [w172]
              tunnel: [w172] -> w169
              tunnel: w164 -> [w171]
              tunnel: [w171] -> w167
              tunnel: w169 -> [w177]
              tunnel: [w177] -> w168
              tunnel: w167 -> [w176]
              tunnel: [w176] -> w166
              tunnel: w170 -> [w179]
              tunnel: w168 -> [w183]
              tunnel: w166 -> [w182]
              tunnel: [w181] -> w163
              tunnel: [w180] -> w162
              tunnel: [w179] -> w161
              tunnel: w163 -> [w204]
              tunnel: w162 -> [w203]
              tunnel: w161 -> [w205]
              tunnel: [w202] -> w160
              tunnel: [w201] -> w159
              frame #0 {
                n190 = case shown="False" w173 {
                  frame False {
                    w174 = T2."Enabled" ("Disabled")
                    n191 = property on="btn_set" class="Bool (strict)"("DisabledEnum"=w174) -> ()  [unwired: 2 in, 2 out]
                    n192 = property on="btn_get" class="Bool (strict)"("DisabledEnum"=w174) -> ()  [unwired: 2 in, 2 out]
                    n193 = property on="num_pulse_samples" class="DigNum (strict)"("DisabledEnum"=w174) -> ()  [unwired: 2 in, 2 out]
                    n194 = property on="num_pulse_freq" class="DigNum (strict)"("DisabledEnum"=w174) -> ()  [unwired: 2 in, 2 out]
                    n195 = property on="num_sensor_sam_per_cycle" class="DigNum (strict)"("DisabledEnum"=w174) -> ()  [unwired: 2 in, 2 out]
                    n196 = property on="num_senor_read_samples" class="DigNum (strict)"("DisabledEnum"=w174) -> ()  [unwired: 2 in, 2 out]
                    n197 = property on="num_pulse_max_val" class="DigNum (strict)"("DisabledEnum"=w174) -> ()  [unwired: 2 in, 2 out]
                    n198 = property on="num_pulse_min_val" class="DigNum (strict)"("DisabledEnum"=w174) -> ()  [unwired: 2 in, 2 out]
                    n199 = property on="num_pulse_dutyc" class="DigNum (strict)"("DisabledEnum"=w174) -> ()  [unwired: 2 in, 2 out]
                    n200 = property on="cbx_sensor_sam_rate" class="CmbBox"("DisabledEnum"=w174) -> ()  [unwired: 2 in, 2 out]
                    n201 = property on="cbx_pulse_type" class="CmbBox"("DisabledEnum"=w174) -> ()  [unwired: 2 in, 2 out]
                  }
                  frame True {
                    w175 = T2."Disabled and Grayed Out" ("Disabled")
                    n202 = property on="btn_get" class="Bool (strict)"("DisabledEnum"=w175) -> ()  [unwired: 2 in, 2 out]
                    n203 = property on="btn_set" class="Bool (strict)"("DisabledEnum"=w175) -> ()  [unwired: 2 in, 2 out]
                    n204 = property on="num_senor_read_samples" class="DigNum (strict)"("DisabledEnum"=w175) -> ()  [unwired: 2 in, 2 out]
                    n205 = property on="num_sensor_sam_per_cycle" class="DigNum (strict)"("DisabledEnum"=w175) -> ()  [unwired: 2 in, 2 out]
                    n206 = property on="cbx_sensor_sam_rate" class="CmbBox"("DisabledEnum"=w175) -> ()  [unwired: 2 in, 2 out]
                    n207 = property on="cbx_pulse_type" class="CmbBox"("DisabledEnum"=w175) -> ()  [unwired: 2 in, 2 out]
                    n208 = property on="num_pulse_min_val" class="DigNum (strict)"("DisabledEnum"=w175) -> ()  [unwired: 2 in, 2 out]
                    n209 = property on="num_pulse_max_val" class="DigNum (strict)"("DisabledEnum"=w175) -> ()  [unwired: 2 in, 2 out]
                    n210 = property on="num_pulse_dutyc" class="DigNum (strict)"("DisabledEnum"=w175) -> ()  [unwired: 2 in, 2 out]
                    n211 = property on="num_pulse_freq" class="DigNum (strict)"("DisabledEnum"=w175) -> ()  [unwired: 2 in, 2 out]
                    n212 = property on="num_pulse_samples" class="DigNum (strict)"("DisabledEnum"=w175) -> ()  [unwired: 2 in, 2 out]
                  }
                }
              }
              frame #1 {
                n213 = local write "has_response"(FALSE ("IS_RESPONSE")) -> ()
              }
              frame #2 {
                n214 = case shown="True" w179 {
                  tunnel: [w189 w197] -> w184
                  frame False {
                    n215 = local read "CMD_RUN_STOP"() -> (w190:string)
                    n216 = local read "CMD_ID_RUN"() -> (w191:string)
                    n217 = Initialize Array(u8 0 ("element"), 32 ("dimension size")) -> (w186:u8[])
                    n218 = Concatenate Strings(w191, w190) -> (w192:string)
                    n219 = Byte Array To String(unsigned byte array=w186) -> (string=w185:string)
                    n220 = Concatenate Strings(w192, w185) -> (w189:string)
                  }
                  frame True {
                    n221 = local read "CMD_RUN_START"() -> (w199:string)
                    n222 = local read "CMD_ID_RUN"() -> (w200:string)
                    n223 = Initialize Array(u8 0 ("element"), 32 ("dimension size")) -> (w194:u8[])
                    n224 = Concatenate Strings(w200, w199) -> (w198:string)
                    n225 = Byte Array To String(unsigned byte array=w194) -> (string=w193:string)
                    n226 = Concatenate Strings(w198, w193) -> (w197:string)
                  }
                }
                n227 = VISA Write(VISA resource name=w183, write buffer=w184, error in (no error)=w182) -> (VISA resource name out=w181:refnum<visa-resource-name>, error out=w180:errorcluster)  [unwired: 1 out]
                n228 = local write item#35(w184) -> ()
              }
              frame #3 {
                n229 = case shown="False" w205 {
                  tunnel: w204 -> [w211 w220]
                  tunnel: w203 -> [w209 w219]
                  tunnel: [w207 w220] -> w202
                  tunnel: [w206 w219] -> w201
                  frame False {
                    n230 = flat-sequence {
                      tunnel: w211 -> [w213]
                      tunnel: [w213] -> w210
                      tunnel: w209 -> [w212]
                      tunnel: [w212] -> w208
                      tunnel: w210 -> [w218]
                      tunnel: w208 -> [w217]
                      tunnel: [w216] -> w207
                      tunnel: [w215] -> w206
                      frame #0 {
                        # "Wait until the Firmware stop"
                        n231 = Wait (ms)(milliseconds to wait=u32 100) -> ()  [unwired: 1 out]
                      }
                      frame #1 {
                        # "Flush any data in the read buffer\nof VISA to be ready for new reading data."
                        n232 = VISA Flush I/O Buffer(VISA resource name=w218, error in (no error)=w217) -> (VISA resource name out=w216:refnum<visa-resource-name>, error out=w215:errorcluster)  [unwired: 1 in]
                      }
                    }
                  }
                  frame True {
                  }
                }
              }
            }
          }
          event "btn_set": Value Change {
            n233 = event-data() -> ("NewVal"=w225:bool)  [unwired: 1 in]
            n234 = case shown="True" w225 {
              tunnel: w222 -> [w227 w231]
              tunnel: w221 -> [w226 w230]
              tunnel: [w227 w229] -> w224
              tunnel: [w226 w228] -> w223
              frame False {
              }
              frame True {
                n235 = local read "num_pulse_samples"() -> (w232:u32)
                n236 = local read "num_pulse_freq"() -> (w234:u32)
                n237 = local read "TIM_FREQ"() -> (w235:u32)
                n238 = Multiply(x=w234, y=w232) -> (x*y=w233:u32)
                n239 = Quotient & Remainder(x=w235, y=w233) -> (x-y*floor(x/y)=w237:u32)  [unwired: 1 out]
                n240 = Equal To 0?(x=w237) -> (x = 0?=w236:bool)
                n241 = case shown="True" w236 {
                  tunnel: w231 -> [w239 w249]
                  tunnel: w230 -> [w238 w247]
                  tunnel: [w239 w245] -> w229
                  tunnel: [w238 w244] -> w228
                  frame False {
                    n242 = local read "TIM_FREQ"() -> (w240:u32)
                    n243 = Number To Decimal String(number=w240) -> (decimal integer string=w242:string)  [unwired: 1 in]
                    n244 = Concatenate Strings("The product of frequency and samples of the pulse must be a divisor of the timer frequency  " ("string"), w242) -> (w241:string)
                    n245 = One Button Dialog(message=w241) -> ()  [unwired: 1 in, 1 out]
                  }
                  frame True {
                    n246 = flat-sequence {
                      tunnel: w249 -> [w251]
                      tunnel: [w251] -> w248
                      tunnel: w247 -> [w250]
                      tunnel: [w250] -> w246
                      tunnel: w248 -> [w256]
                      tunnel: w246 -> [w255]
                      tunnel: [w254] -> w245
                      tunnel: [w253] -> w244
                      frame #0 {
                        n247 = local write "has_response"(FALSE ("IS_RESPONSE")) -> ()
                      }
                      frame #1 {
                        w264 = FALSE ("prepend array or string size? (T)")
                        w263 = T3."big-endian, network order" ("byte order (0:big-endian, network order)")
                        n248 = local read "sam_rates"() -> (w272:cluster{u32, u32, dbl}[])
                        n249 = local read "num_pulse_max_val"() -> (w301:dbl)
                        n250 = local read "cbx_pulse_type"() -> (w303:string)
                        n251 = for {
                          tunnel: w272 -> [w309] mode=indexing
                          tunnel: [w308] -> w271 mode=indexing
                          tunnel: [w307] -> w270 mode=indexing
                          n252 = Unbundle(w309) -> (w307:u32, w308:dbl)  [unwired: 1 out]
                        }
                        n253 = local read "num_pulse_min_val"() -> (w299:dbl)
                        n254 = local read "cbx_sensor_sam_rate_sel_idx"() -> (w257:u32)
                        n255 = local read "num_senor_read_samples"() -> (w282:u32)
                        n256 = local read "num_pulse_samples"() -> (w277:u32)
                        n257 = Decimal String To Number(string=w303) -> (number=w304:i32)  [unwired: 2 in, 1 out]
                        n258 = local read "num_pulse_dutyc"() -> (w279:u32)
                        n259 = local read "num_pulse_freq"() -> (w280:u32)
                        n260 = Multiply(x=w301, y=1000.0) -> (x*y=w300:dbl)
                        n261 = Initialize Array(w304, 1 ("dimension size")) -> (w305:i32[])
                        n262 = local read "CMD_ID_SET"() -> (w289:string)
                        n263 = Multiply(x=w299, y=1000.0) -> (x*y=w297:dbl)
                        n264 = Index Array(array=w270, index=w257) -> (element=w269:u32)
                        n265 = Index Array(array=w271, index=w257) -> (element=w268:dbl)
                        n266 = To Unsigned Long Integer(number=w280) -> (unsigned 32bit integer=w281:u32)
                        n267 = To Unsigned Long Integer(number=w279) -> (unsigned 32bit integer=w278:u32)
                        n268 = To Unsigned Long Integer(number=w300) -> (unsigned 32bit integer=w302:u32)
                        n269 = To Unsigned Long Integer(number=w277) -> (unsigned 32bit integer=w276:u32)
                        n270 = To Unsigned Long Integer(number=w282) -> (unsigned 32bit integer=w273:u32)
                        n271 = Byte Array To String(unsigned byte array=w305) -> (string=w306:string)
                        n272 = Concatenate Strings(w289, w306) -> (w291:string)
                        n273 = Flatten To String(anything=w281, prepend array or string size? (T)=w264, byte order (0:big-endian, network order)=w263) -> (data string=w290:string)  [unwired: 1 in, 2 out]
                        n274 = Flatten To String(anything=w278, prepend array or string size? (T)=w264, byte order (0:big-endian, network order)=w263) -> (data string=w294:string)  [unwired: 1 in, 2 out]
                        n275 = Flatten To String(anything=w302, prepend array or string size? (T)=w264, byte order (0:big-endian, network order)=w263) -> (data string=w288:string)  [unwired: 1 in, 2 out]
                        n276 = Flatten To String(anything=w276, prepend array or string size? (T)=w264, byte order (0:big-endian, network order)=w263) -> (data string=w283:string)  [unwired: 1 in, 2 out]
                        n277 = Flatten To String(anything=w269, prepend array or string size? (T)=w264, byte order (0:big-endian, network order)=w263) -> (data string=w260:string)  [unwired: 1 in, 2 out]
                        n278 = Flatten To String(anything=w273, prepend array or string size? (T)=w264, byte order (0:big-endian, network order)=w263) -> (data string=w275:string)  [unwired: 1 in, 2 out]
                        n279 = To Unsigned Long Integer(number=w297) -> (unsigned 32bit integer=w298:u32)
                        n280 = Multiply(x=w268, y=10.0) -> (x*y=w266:dbl)
                        n281 = Concatenate Strings(w291, w290) -> (w292:string)
                        n282 = Flatten To String(anything=w298, prepend array or string size? (T)=w264, byte order (0:big-endian, network order)=w263) -> (data string=w296:string)  [unwired: 1 in, 2 out]
                        n283 = To Unsigned Long Integer(number=w266) -> (unsigned 32bit integer=w265:u32)
                        n284 = Concatenate Strings(w292, w294) -> (w293:string)
                        n285 = Flatten To String(anything=w265, prepend array or string size? (T)=w264, byte order (0:big-endian, network order)=w263) -> (data string=w261:string)  [unwired: 1 in, 2 out]
                        n286 = Concatenate Strings(w293, w288) -> (w295:string)
                        n287 = Concatenate Strings(w295, w296) -> (w284:string)
                        n288 = Concatenate Strings(w284, w283) -> (w259:string)
                        n289 = Concatenate Strings(w259, w260) -> (w262:string)
                        n290 = Concatenate Strings(w262, w261) -> (w258:string)
                        n291 = Concatenate Strings(w258, w275) -> (w274:string)
                        n292 = VISA Write(VISA resource name=w256, write buffer=w274, error in (no error)=w255) -> (VISA resource name out=w254:refnum<visa-resource-name>, error out=w253:errorcluster)  [unwired: 1 out]
                        n293 = local write item#35(w274) -> ()
                      }
                    }
                  }
                }
              }
            }
          }
          event "btn_get": Value Change {
            n294 = event-data() -> ("NewVal"=w314:bool)  [unwired: 1 in]
            n295 = case shown="True" w314 {
              tunnel: w312 -> [w316 w322]
              tunnel: w313 -> [w315 w320]
              tunnel: [w316 w318] -> w311
              tunnel: [w315 w317] -> w310
              frame False {
              }
              frame True {
                n296 = flat-sequence {
                  tunnel: w322 -> [w324]
                  tunnel: [w324] -> w321
                  tunnel: w320 -> [w323]
                  tunnel: [w323] -> w319
                  tunnel: w321 -> [w329]
                  tunnel: w319 -> [w328]
                  tunnel: [w327] -> w318
                  tunnel: [w326] -> w317
                  frame #0 {
                    n297 = local write "has_response"(TRUE ("IS_RESPONSE")) -> ()
                  }
                  frame #1 {
                    n298 = Initialize Array(u8 0 ("element"), 33 ("dimension size")) -> (w331:u8[])
                    n299 = local read "CMD_ID_GET"() -> (w335:string)
                    n300 = Byte Array To String(unsigned byte array=w331) -> (string=w330:string)
                    n301 = Concatenate Strings(w335, w330) -> (w334:string)
                    n302 = VISA Write(VISA resource name=w329, write buffer=w334, error in (no error)=w328) -> (VISA resource name out=w327:refnum<visa-resource-name>, error out=w326:errorcluster)  [unwired: 1 out]
                    n303 = local write item#35(w334) -> ()
                  }
                }
              }
            }
          }
          event "num_pulse_freq", "cbx_sensor_sam_rate": Value Change {
            n304 = event-data() -> ()  [unwired: 1 in, 1 out]
            n305 = property on="cbx_sensor_sam_rate" class="CmbBox"() -> ("Strings[]"=w339:string[])  [unwired: 2 in, 2 out]
            n306 = local read "num_pulse_freq"() -> (w336:u32)
            n307 = Greater Than 0?(x=w336) -> (x > 0?=w337:bool)
            n308 = while {
              tunnel: w339 -> [w344] mode=indexing
              tunnel: [w341] -> w340
              i -> [w341]
              stop <- w342 stop-if-true
              n309 = local read "cbx_sensor_sam_rate"() -> (w343:string)
              n310 = Equal?(x=w344, y=w343) -> (x = y?=w342:bool)
            }
            "cbx_sensor_sam_rate_sel_idx" <- w340
            n311 = case shown="True" w337 {
              tunnel: [0 w350] -> w338
              frame False {
              }
              frame True {
                n312 = local read "cbx_sensor_sam_rate"() -> (w346:string)
                n313 = local read "num_pulse_freq"() -> (w348:u32)
                n314 = Decimal String To Number(string=w346) -> (number=w347:i32)  [unwired: 2 in, 1 out]
                n315 = Divide(x=w347, y=w348) -> (x/y=w349:dbl)
                n316 = To Unsigned Long Integer(number=w349) -> (unsigned 32bit integer=w350:u32)
              }
            }
            n317 = local write "num_sensor_sam_per_cycle"(w338) -> ()
          }
        }
      }
      n318 = VISA Close(VISA resource name=w134, error in (no error)=w135) -> ()  [unwired: 1 out]
      n319 = VISA Close(VISA resource name=w129, error in (no error)=w128) -> ()  [unwired: 1 out]
    }
  }
